vi "Agilent Valve Control.vi"(0 "Station In":string, 1 "Agilent Channels In":T2[](array[typedef])=[{"Channel"="301", "Station"="1", "Label"="Water Valve", "Agilent Station"="2"}, {"Channel"="302", "Station"="2", "Label"="Water Valve", "Agilent Station"="2"}, {"Channel"="303", "Station"="3", "Label"="Water Valve", "Agilent Station"="2"}, {"Channel"="304", "Station"="4", "Label"="Water Valve", "Agilent Station"="2"}, {"Channel"="305", "Station"="5", "Label"="Water Valve", "Agilent Station"="2"}, {"Channel"="306", "Station"="6", "Label"="Water Valve", "Agilent Station"="2"}, {"Channel"="307", "Station"="7", "Label"="Water Valve", "Agilent Station"="2"}, {"Channel"="308", "Station"="8", "Label"="Water Valve", "Agilent Station"="2"}, {"Channel"="309", "Station"="9", "Label"="Water Valve", "Agilent Station"="2"}, {"Channel"="310", "Station"="10", "Label"="Water Valve", "Agilent Station"="2"}, {"Channel"="311", "Station"="11", "Label"="Water Valve", "Agilent Station"="2"}, {"Channel"="312", "Station"="12", "Label"="Water Valve", "Agilent Station"="2"}, {"Channel"="313", "Station"="13", "Label"="Water Valve", "Agilent Station"="2"}, {"Channel"="314", "Station"="14", "Label"="Water Valve", "Agilent Station"="2"}, {"Channel"="315", "Station"="15", "Label"="Water Valve", "Agilent Station"="2"}, {"Channel"="316", "Station"="16", "Label"="Water Valve", "Agilent Station"="2"}, {"Channel"="317", "Station"="17", "Label"="Water Valve", "Agilent Station"="2"}, {"Channel"="318", "Station"="18", "Label"="Water Valve", "Agilent Station"="2"}, {"Channel"="319", "Station"="19", "Label"="Water Valve", "Agilent Station"="2"}, {"Channel"="320", "Station"="20", "Label"="Water Valve", "Agilent Station"="2"}, {"Channel"="101", "Station"="21", "Label"="Water Valve", "Agilent Station"="3"}, {"Channel"="102", "Station"="22", "Label"="Water Valve", "Agilent Station"="3"}, {"Channel"="103", "Station"="23", "Label"="Water Valve", "Agilent Station"="3"}, {"Channel"="104", "Station"="24", "Label"="Water Valve", "Agilent Station"="3"}, {"Channel"="105", "Station"="25", "Label"="Water Valve", "Agilent Station"="3"}, {"Channel"="106", "Station"="26", "Label"="Water Valve", "Agilent Station"="3"}, {"Channel"="107", "Station"="27", "Label"="Water Valve", "Agilent Station"="3"}, {"Channel"="108", "Station"="28", "Label"="Water Valve", "Agilent Station"="3"}, {"Channel"="109", "Station"="29", "Label"="Water Valve", "Agilent Station"="3"}, {"Channel"="110", "Station"="30", "Label"="Water Valve", "Agilent Station"="3"}, {"Channel"="111", "Station"="31", "Label"="Water Valve", "Agilent Station"="3"}, {"Channel"="112", "Station"="32", "Label"="Water Valve", "Agilent Station"="3"}, {"Channel"="101", "Station"="33", "Label"="Water Valve", "Agilent Station"="5"}, {"Channel"="102", "Station"="34", "Label"="Water Valve", "Agilent Station"="5"}, {"Channel"="103", "Station"="35", "Label"="Water Valve", "Agilent Station"="5"}, {"Channel"="104", "Station"="36", "Label"="Water Valve", "Agilent Station"="5"}, {"Channel"="105", "Station"="37", "Label"="Water Valve", "Agilent Station"="5"}, {"Channel"="106", "Station"="38", "Label"="Water Valve", "Agilent Station"="5"}, {"Channel"="107", "Station"="39", "Label"="Water Valve", "Agilent Station"="5"}, {"Channel"="108", "Station"="40", "Label"="Water Valve", "Agilent Station"="5"}, {"Channel"="109", "Station"="41", "Label"="Water Valve", "Agilent Station"="5"}, {"Channel"="110", "Station"="42", "Label"="Water Valve", "Agilent Station"="5"}, {"Channel"="111", "Station"="43", "Label"="Water Valve", "Agilent Station"="5"}, {"Channel"="112", "Station"="44", "Label"="Water Valve", "Agilent Station"="5"}, {"Channel"="113", "Station"="45", "Label"="Water Valve", "Agilent Station"="5"}, {"Channel"="114", "Station"="46", "Label"="Water Valve", "Agilent Station"="5"}, {"Channel"="115", "Station"="47", "Label"="Water Valve", "Agilent Station"="5"}, {"Channel"="116", "Station"="48", "Label"="Water Valve", "Agilent Station"="5"}, {"Channel"="117", "Station"="49", "Label"="Water Valve", "Agilent Station"="5"}, {"Channel"="118", "Station"="50", "Label"="Water Valve", "Agilent Station"="5"}, {"Channel"="119", "Station"="51", "Label"="Water Valve", "Agilent Station"="5"}, {"Channel"="120", "Station"="52", "Label"="Water Valve", "Agilent Station"="5"}, {"Channel"="201", "Station"="53", "Label"="Water Valve", "Agilent Station"="5"}, {"Channel"="202", "Station"="54", "Label"="Water Valve", "Agilent Station"="5"}, {"Channel"="203", "Station"="55", "Label"="Water Valve", "Agilent Station"="5"}, {"Channel"="204", "Station"="56", "Label"="Water Valve", "Agilent Station"="5"}], 2 "Agilent":T1, 5 "Open/Close (F:Close)":bool, 11 "error in (no error)":errorcluster) -> (4 "Channel State?":string, 6 "Success":bool, 15 "error out":errorcluster)   [LabVIEW 2012]
uses:
  Agilent Channel Definition.ctl
  Drivers/Agilent 34970/Agilent 34970.lvlib
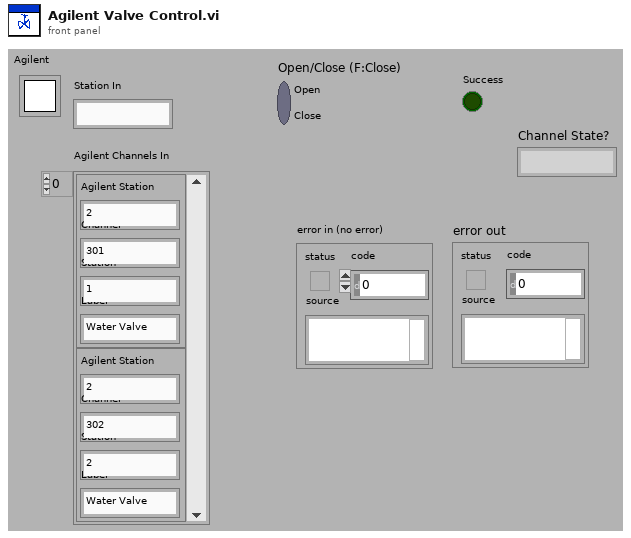
[diagram p1: front panel]
types:
  T1 = typedef "Semaphore RefNum" = refnum<k1>
  T2 = typedef "Agilent Channel Definition.ctl" = cluster{"Channel":string, "Station":string, "Label":string, "Agilent Station":string}
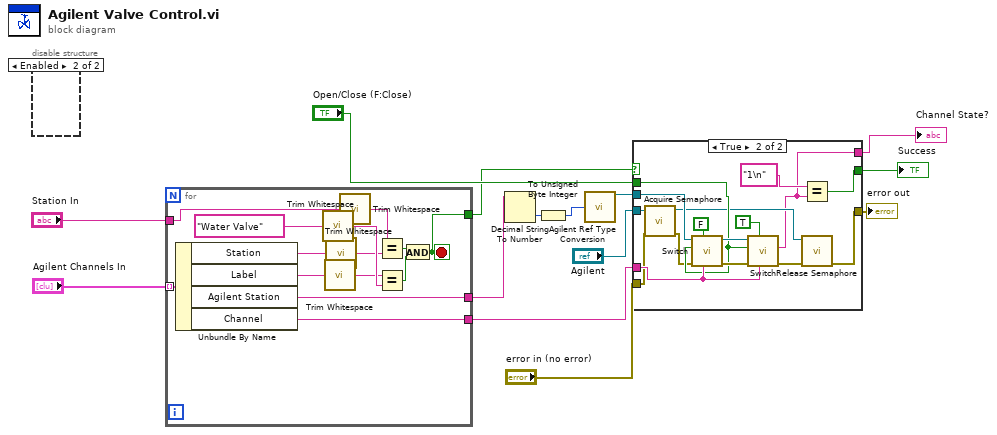
[diagram p0: block diagram]
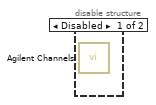
[diagram p2: hidden frame]
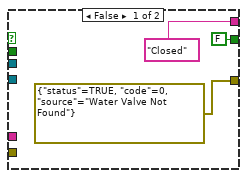
[diagram p3: hidden frame]
diagram:
  n1 = disable-structure shown="Enabled" {
    frame Disabled {
      n2 = call "Agilent Channels.vi"() -> ()  [unwired: 9 in, 7 out]
    }
    frame Enabled {
    }
  }
  n3 = for {
    tunnel: "Agilent Channels In" -> [w28] mode=indexing
    tunnel: "Station In" -> [w19]
    tunnel: [w25] -> w13
    tunnel: [w24] -> w6
    tunnel: [w23] -> w5
    stop <- w23 stop-if-true
    n4 = Unbundle By Name(w28) -> ("Station"=w16:string, "Label"=w22:string, "Agilent Station"=w25:string, "Channel"=w24:string)
    n5 = call <vilib>:"Trim Whitespace.vi"("string"="Water Valve" ("y")) -> ("trimmed string"=w20:string)  [unwired: 1 in]
    n6 = call <vilib>:"Trim Whitespace.vi"("string"=w22) -> ("trimmed string"=w17:string)  [unwired: 1 in]
    n7 = call <vilib>:"Trim Whitespace.vi"("string"=w16) -> ("trimmed string"=w15:string)  [unwired: 1 in]
    n8 = call <vilib>:"Trim Whitespace.vi"("string"=w19) -> ("trimmed string"=w18:string)  [unwired: 1 in]
    n9 = Equal?(x=w18, y=w15) -> (x = y?=w26:bool)
    n10 = Equal?(x=w17, y=w20) -> (x = y?=w27:bool)
    n11 = And(x=w26, y=w27) -> (x .and. y?=w23:bool)
  }
  n12 = Decimal String To Number(string=w13) -> (number=w12:i32)  [unwired: 2 in, 1 out]
  n13 = To Unsigned Byte Integer(number=w12) -> (unsigned 8bit integer=w11:u8)
  n14 = call "Agilent Ref Type Conversion.vi"("Agilent Ref"=w11) -> ("VISA resource name"=w10:refnum<visa-resource-name>)  [unwired: 14 in]
  n15 = case shown="True" w5 {
    tunnel: w10 -> [_ w47]
    tunnel: "Open/Close (F:Close)" -> [_ w41]
    tunnel: "error in (no error)" -> [_ w38]
    tunnel: [errorcluster {"status"=TRUE, "code"=0, "source"="Water Valve Not Found"} ("error out") w35] -> w7
    tunnel: w6 -> [_ w42]
    tunnel: [FALSE w43] -> w4
    tunnel: "Agilent" -> [_ w39]
    tunnel: ["Closed" w32] -> w1
    frame False {
    }
    frame True {
      n16 = call <vilib>:"Acquire Semaphore.vi"("error in (no error)"=w38, "semaphore"=w39) -> ("error out"=w37:errorcluster, "semaphore out"=w34:T1)  [unwired: 3 in, 1 out]
      n17 = call "Switch.vi"("Channel List(empty)"=w42, "Set/Check (F:Set)"=FALSE, "error in (no error)"=w37, "Open/Close (F:Close)"=w41, "VISA Resource Name"=w47) -> ("error out"=w46:errorcluster, "VISA Resource Name Out"=w45:refnum<visa-resource-name>)  [unwired: 4 in, 1 out]
      n18 = call "Switch.vi"("Channel List(empty)"=w42, "Set/Check (F:Set)"=TRUE, "error in (no error)"=w46, "Open/Close (F:Close)"=w41, "VISA Resource Name"=w45) -> ("error out"=w36:errorcluster, "Channel State?"=w32:string)  [unwired: 4 in, 1 out]
      n19 = Equal?(x="1\n" ("Channel State?"), y=w32) -> (x = y?=w43:bool)
      n20 = call <vilib>:"Release Semaphore.vi"("error in (no error)"=w36, "semaphore"=w34) -> ("error out"=w35:errorcluster)  [unwired: 4 in, 1 out]
    }
  }
  "error out" <- w7
  "Success" <- w4
  "Channel State?" <- w1
